vi "IVSweep.vi"(0 "VISA Refnum in":refnum<visa-resource-name>, 3 "Source Measure Unit Channel (0: Channel A)":i32(ring) items=["Channel A", "Channel B"], 5 "Sweep List (V)":dbl[](array[numeric])) -> (14 "Current (A)":dbl[](array[numeric]), 19 "error out":errorcluster)   [LabVIEW 2020]
uses:
  Keithley 2600 Series/Keithley 2600 Series.lvlib
panel:
  in  "Script":string="smua.reset()\nsmua.source.func = smua.OUTPUT_DCAMPS\nsmua.source.rangei = 10e-3\nsmua.source.leveli = 10e-3\nsmua.source.limitv = 10 \n\nvoltages={}\n\n"
  in  "Delay Time":dbl=0.5
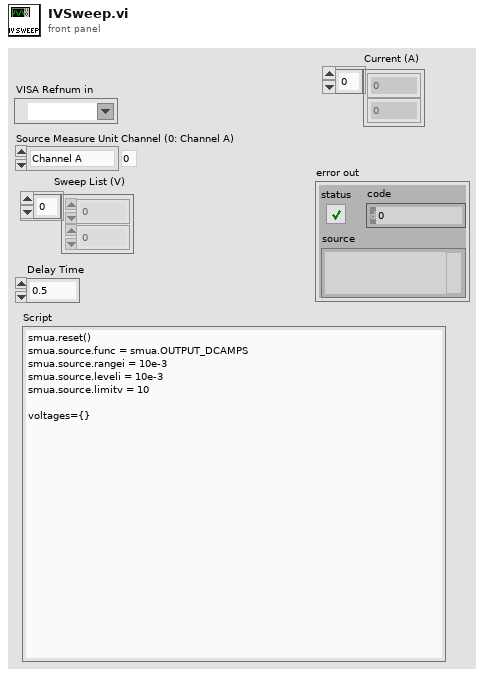
[diagram p1: front panel]
types:
  T1 = enum16{"Native", "Native Command Line", "UNIX", "Macintosh", "DOS"}
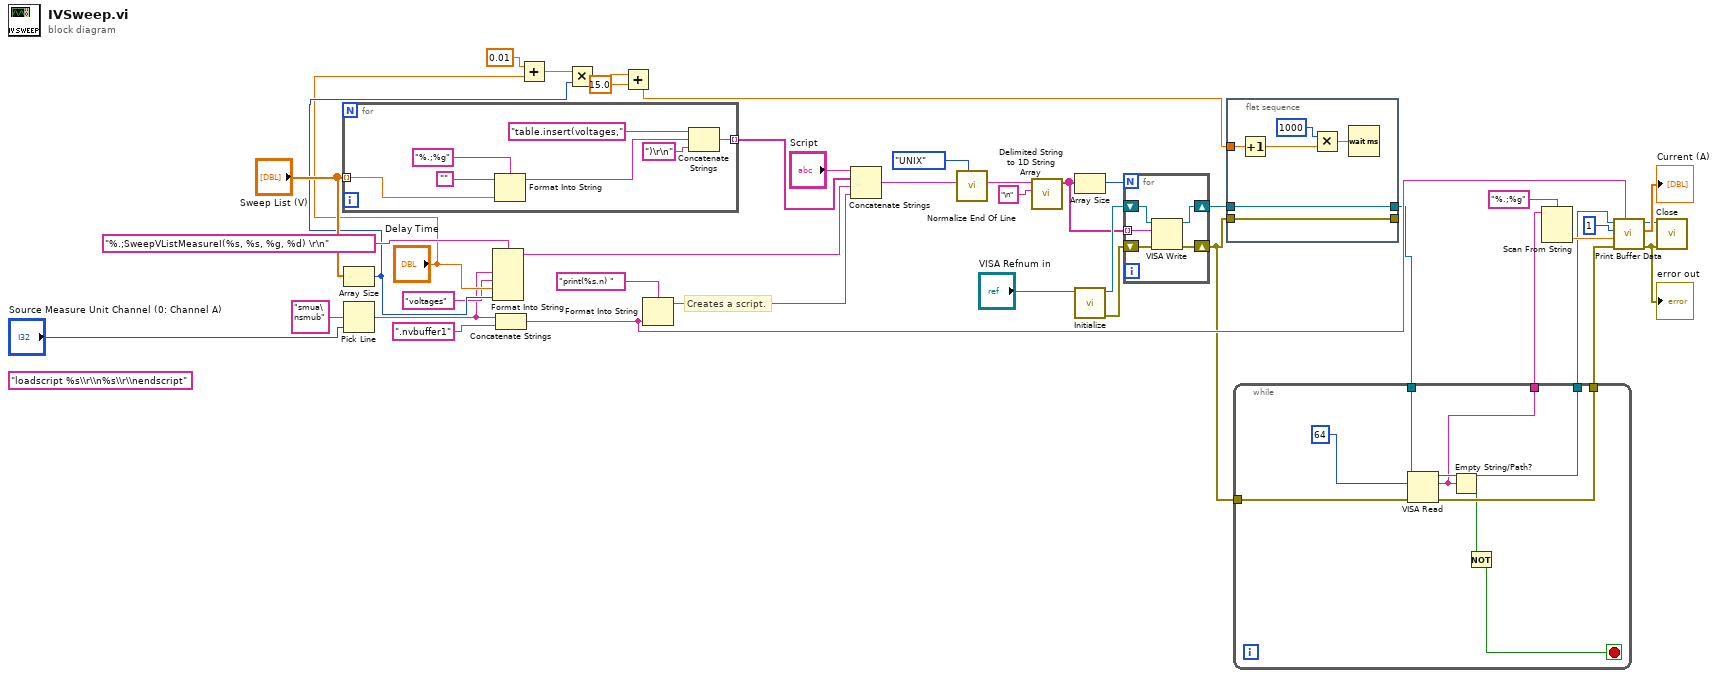
[diagram p0: block diagram]
diagram:
  (unwired) "loadscript %s\\r\\n%s\\r\\nendscript"
  # "Creates a script."
  n1 = for {
    tunnel: "Sweep List (V)" -> [w48] mode=indexing
    tunnel: [w43] -> w30 mode=indexing
    n2 = Format Into String(format string="%.;%g", initial string="", w48) -> (resulting string=w45:string)  [unwired: 1 in, 1 out]
    n3 = Concatenate Strings("table.insert(voltages," ("string"), w45, ")\r\n" ("string")) -> (w43:string)
  }
  n4 = Array Size(array="Sweep List (V)") -> (size(s)=w34:i32)
  n5 = Pick Line(multi-line string="smua\nsmub", line index="Source Measure Unit Channel (0: Channel A)") -> (output string=w27:string)  [unwired: 1 in]
  n6 = Format Into String(format string="%.;SweepVListMeasureI(%s, %s, %g, %d) \r\n", w27, "voltages" ("input 2"), "Delay Time", w34) -> (resulting string=w31:string)  [unwired: 2 in, 1 out]
  n7 = Concatenate Strings(w27, ".nvbuffer1" ("string")) -> (w18:string)
  n8 = Add(x=0.01, y="Delay Time") -> (x+y=w37:dbl)
  n9 = Multiply(x=w37, y=w34) -> (x*y=w20:dbl)
  n10 = Add(x=w20, y=15.0) -> (x+y=w2:dbl)
  n11 = Format Into String(format string="print(%s.n) ", w18) -> (resulting string=w8:string)  [unwired: 2 in, 1 out]
  n12 = Concatenate Strings("Script", w30, w31, w8) -> (w17:string)
  n13 = call <vilib>:"Normalize End Of Line.vi"("end of line (Native)"=T1."UNIX", "string in"=w17) -> ("string out"=w10:string)  [unwired: 6 in]
  n14 = call <vilib>:"Delimited String to 1D String Array.vi"("delimiter"="\n", "delimited string"=w10) -> ("string array"=w13:string[])  [unwired: 9 in]
  n15 = Array Size(array=w13) -> (size(s)=w12:i32)
  n16 = call "Initialize.vi"("VISA resource name"="VISA Refnum in") -> ("error out"=w15:errorcluster, "VISA resource name out"=w14:refnum<visa-resource-name>)  [unwired: 9 in]
  n17 = for {
    N: w12 -> [_]
    shift-right: [w49] -> w7
    shift-left: w15 -> [w53]
    shift-right: [w50] -> w11
    shift-left: w14 -> [w52]
    tunnel: w13 -> [w51] mode=indexing
    n18 = VISA Write(VISA resource name=w52, write buffer=w51, error in (no error)=w53) -> (VISA resource name out=w50:refnum<visa-resource-name>, error out=w49:errorcluster)  [unwired: 1 out]
  }
  n19 = flat-sequence {
    tunnel: w11 -> [w59]
    tunnel: [w59] -> w6
    tunnel: w2 -> [w58]
    tunnel: w7 -> [w54]
    tunnel: [w54] -> _
    frame #0 {
      n20 = Increment(x=w58) -> (x+1=w57:dbl)
      n21 = Multiply(x=1000, y=w57) -> (x*y=w55:dbl)
      n22 = Wait (ms)(milliseconds to wait=w55) -> ()  [unwired: 1 out]
    }
  }
  n23 = while {
    tunnel: w7 -> [w67]
    tunnel: w6 -> [w66]
    tunnel: [w65] -> w5
    tunnel: [w63] -> w4
    tunnel: [w64] -> w3
    stop <- w61 stop-if-true
    n24 = VISA Read(VISA resource name=w66, byte count=u32 64, error in (no error)=w67) -> (VISA resource name out=w64:refnum<visa-resource-name>, read buffer=w63:string, error out=w65:errorcluster)  [unwired: 1 out]
    n25 = Empty String/Path?(string/path=w63) -> (empty?=w62:bool)
    n26 = Not(x=w62) -> (.not. x?=w61:bool)
  }
  n27 = Scan From String(format string="%.;%g", input string=w4) -> (output 1=w24:dbl)  [unwired: 3 in, 3 out]
  n28 = call "Print Buffer Data.vi"("Reading Buffer (smua.nvbuffer1)"=w18, "error in (no error)"=w5, "End Index (1)"=w24, "Start Index (1)"=1 ("Start Index (0)"), "VISA resource name"=w3) -> ("error out"=w21:errorcluster, "Buffer Data"=→"Current (A)":dbl[], "VISA resource name out"=w19:refnum<visa-resource-name>)  [unwired: 4 in]
  "error out" <- w21
  n29 = call "Close.vi"("error in (no error)"=w21, "VISA resource name"=w19) -> ()  [unwired: 9 in, 1 out]
